vi "tcpReadFromZ.vi"(8 "error in (no error)":errorcluster, 9 "Timeout (40000 ms)":i32=40000, 10 "Command sent":string, 11 "connection ID in":refnum<k5>) -> (0 "error out":errorcluster, 2 "receive":string, 3 "connection ID out":refnum<k5>, 4 "time 2 (ms)":u32, 6 "time 1 (ms)":u32)   [LabVIEW 2016]
doc: "Reads a response from the Z system after a Telnet command has been sent. The Z response will start with a status number. The program reads until either a number has been received, or until the timeout (input) is reached. Then, the program continues reading until no more bytes are received for 20 milliseconds; however, if more than 250 characters are received, it reads until an end sequence occurs. The end sequence is two successive end-of-line marks (\\r\\n\\r\\n). Finally, it checks the status number: values outside the range 200-299 are reported as errors."
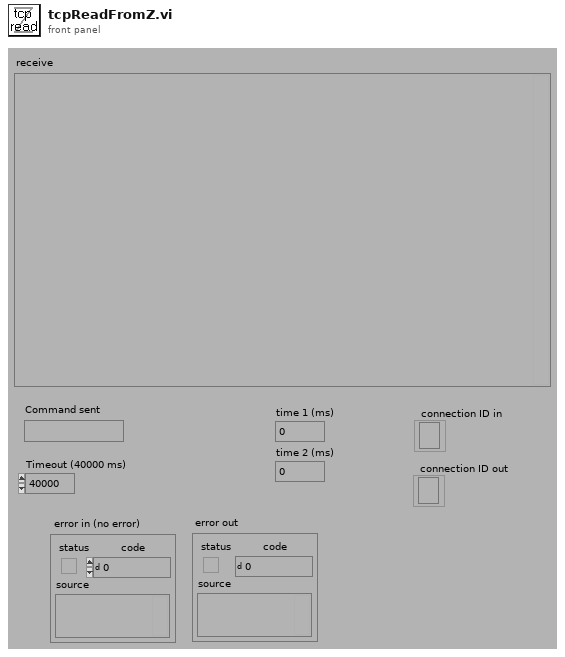
[diagram p1: front panel]
types:
  T1 = enum16{"Standard", "Buffered", "CRLF", "Immediate"}
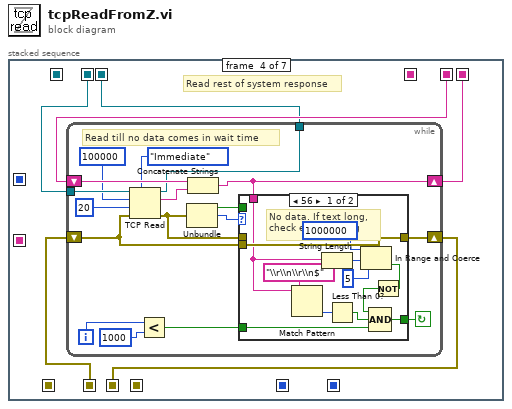
[diagram p0: block diagram]
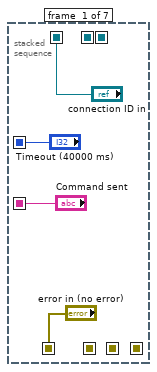
[diagram p2: hidden frame]
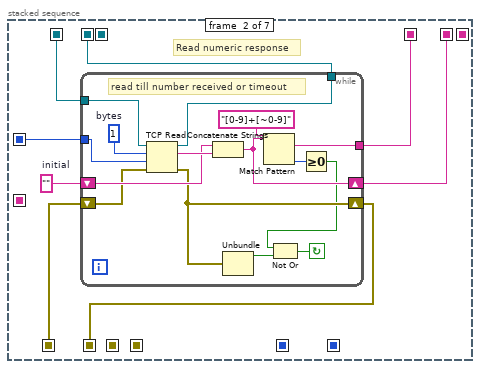
[diagram p3: hidden frame]
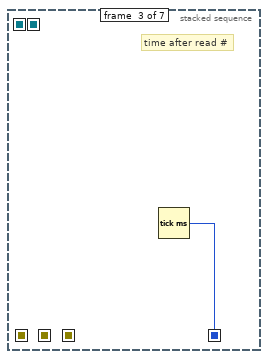
[diagram p4: hidden frame]
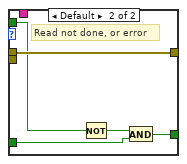
[diagram p5: hidden frame]
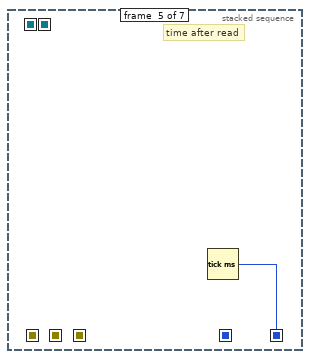
[diagram p6: hidden frame]
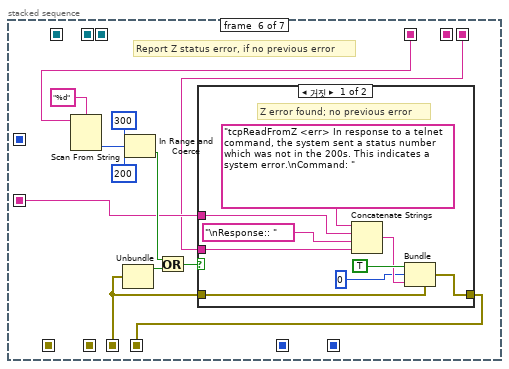
[diagram p7: hidden frame]
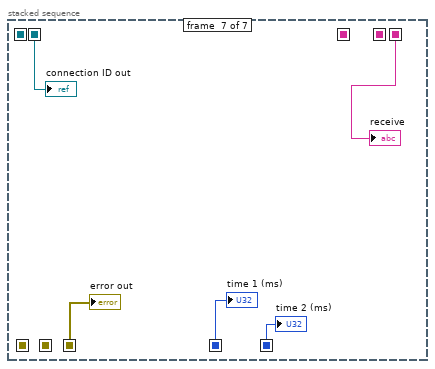
[diagram p9: hidden frame]
diagram:
  n1 = stacked-sequence {
    seq-local: [_ w5 _ _ _ _ _] -> [_ _ _ w33 _ _ _]
    seq-local: ["connection ID in" _ _ _ _ _ _] -> [_ w8 _ _ _ _ _]
    seq-local: ["Timeout (40000 ms)" _ _ _ _ _ _] -> [_ w10 _ _ _ _ _]
    seq-local: ["error in (no error)" _ _ _ _ _ _] -> [_ w7 _ _ _ _ _]
    seq-local: [_ w12 _ _ _ _ _] -> [_ _ _ w34 _ _ _]
    seq-local: [_ w9 _ _ _ _ _] -> [_ _ _ w32 _ _ _]
    seq-local: [_ _ _ w31 _ _ _] -> [_ _ _ _ _ w70 w95]
    seq-local: [_ _ _ w30 _ _ _] -> [_ _ _ _ _ _ w96]
    seq-local: [_ _ _ w29 _ _ _] -> [_ _ _ _ _ w73 _]
    seq-local: [_ _ w28 _ _ _ _] -> [_ _ _ _ _ _ w94]
    seq-local: [_ w6 _ _ _ _ _] -> [_ _ _ _ _ w72 _]
    seq-local: [_ _ _ _ _ w74 _] -> [_ _ _ _ _ _ w93]
    seq-local: ["Command sent" _ _ _ _ _ _] -> [_ _ _ _ _ w71 _]
    seq-local: [_ _ _ _ w69 _ _] -> [_ _ _ _ _ _ w92]
    frame #0 {
    }
    frame #1 {
      w11 = ""  # initial
      # "Read numeric response"
      n2 = while {
        tunnel: [w13] -> w6
        tunnel: w10 -> [w22]
        tunnel: [w23] -> w12
        shift-left: w7 -> [w19]
        shift-right: [w18] -> w5
        tunnel: w8 -> [w27]
        shift-left: w11 -> [w25]
        shift-right: [w21] -> w9
        stop <- w14 continue-if-true
        w24 = 1  # bytes
        # "read till number received or timeout"
        n3 = TCP Read(connection ID=w27, bytes to read=w24, error in (no error)=w19, 9:w22) -> (connection ID out=w23:refnum<k5>, data out=w26:string, error out=w18:errorcluster)  [unwired: 1 in]
        n4 = Concatenate Strings(w25, w26) -> (w21:string)
        n5 = Unbundle(w18) -> ("status"=w15:bool)  [unwired: 2 out]
        n6 = Match Pattern(string=w21, regular expression="[0-9]+[~0-9]") -> (match substring=w13:string, offset past match=w17:i32)  [unwired: 1 in, 2 out]
        n7 = Greater Or Equal To 0?(x=w17) -> (x >= 0?=w16:bool)
        n8 = Not Or(1:w15, 2:w16) -> (0:w14:bool)
      }
    }
    frame #2 {
      # "time after read #"
      n9 = Tick Count (ms)() -> (millisecond timer value=w28:u32)
    }
    frame #3 {
      # "Read rest of system response"
      n10 = while {
        tunnel: [w43] -> w30
        shift-left: w33 -> [w46]
        shift-right: [w44] -> w29
        tunnel: w34 -> [w51]
        shift-left: w32 -> [w49]
        shift-right: [w38] -> w31
        i -> [w37]
        stop <- w42 continue-if-true
        # "Read till no data comes in wait time"
        n11 = TCP Read(connection ID=w51, bytes to read=100000, error in (no error)=w46, 7:T1."Immediate" ("mode (standard)"), 9:20 ("timeout ms (25000)")) -> (connection ID out=w43:refnum<k5>, data out=w50:string, error out=w45:errorcluster)
        n12 = Less?(x=w37, y=1000) -> (x < y?=w35:bool)
        n13 = Unbundle(w45) -> ("status"=w41:bool, "code"=w39:i32)  [unwired: 1 out]
        n14 = Concatenate Strings(w49, w50) -> (w38:string)
        n15 = case shown="56" w39 {
          tunnel: w45 -> [_ w68]
          tunnel: [w63 w68] -> w44
          tunnel: [w62 w64] -> w42
          tunnel: w46 -> [w63 _]
          tunnel: w41 -> [_ w67]
          tunnel: w38 -> [w59 _]
          tunnel: w35 -> [w57 w66]
          frame 56 {
            # "No data. If text long,\ncheck end of string"
            n16 = Match Pattern(string=w59, regular expression="\\r\\n\\r\\n$") -> (offset past match=w61:i32)  [unwired: 1 in, 3 out]
            n17 = String Length(string=w59) -> (length=w56:i32)
            n18 = Less Than 0?(x=w61) -> (x < 0?=w58:bool)
            n19 = In Range and Coerce(upper limit=1000000, x=w56, lower limit=5 ("y")) -> (In Range?=w53:bool)  [unwired: 1 out]
            n20 = Not(x=w53) -> (.not. x?=w52:bool)
            n21 = Compound Arithmetic op=AND(w52, w58, w57) -> (w62:bool)
          }
          frame Default {
            # "Read not done, or error"
            n22 = Not(x=w67) -> (.not. x?=w65:bool)
            n23 = And(x=w65, y=w66) -> (x .and. y?=w64:bool)
          }
        }
      }
    }
    frame #4 {
      # "time after read"
      n24 = Tick Count (ms)() -> (millisecond timer value=w69:u32)
    }
    frame #5 {
      # "Report Z status error, if no previous error"
      n25 = Scan From String(format string="%d" ("Format String"), input string=w72) -> (output 1=w79:i32)  [unwired: 3 in, 3 out]
      n26 = Unbundle(w73) -> ("status"=w76:bool)  [unwired: 2 out]
      n27 = In Range and Coerce(upper limit=i16 300 ("hi"), x=w79, lower limit=i16 200 ("lo")) -> (In Range?=w77:bool)  [unwired: 1 out]
      n28 = Or(x=w77, y=w76) -> (x .or. y?=w75:bool)
      n29 = case shown="거짓" w75 {
        tunnel: [w89 w91] -> w74
        tunnel: w73 -> [w90 w91]
        tunnel: w71 -> [w86 _]
        tunnel: w70 -> [w84 _]
        frame False {
          # "Z error found; no previous error"
          n30 = Concatenate Strings("tcpReadFromZ <err> In response to a telnet command, the system sent a status number which was not in the 200s. This indicates a system error.\nCommand: ", w86, "\nResponse:: " ("Substring"), w84) -> (w83:string)
          n31 = Bundle(cluster=w90, "status"=TRUE ("Bundle Element"), "code"=0 ("Bundle Element"), "source"=w83) -> (w89:errorcluster)
        }
        frame True {
          # "No Z error or previous error"
        }
      }
    }
    frame #6 {
      "connection ID out" <- w96
      "error out" <- w93
      "receive" <- w95
      "time 1 (ms)" <- w94
      "time 2 (ms)" <- w92
    }
  }
